vi "demo_1 Single Run.vi"() -> ()   [LabVIEW 2020]
panel:
  out "mtr status":bool caption="电机运行状态"
  in  "microstepping":u16(ring)=32 caption="细分" items=["1 (200)"=1, "2 (400)"=2, "4 (800)"=4, "8 (1600)"=8, "16 (3200)"=16, "32 (6400)"=32]
  in  "speed":u16 caption="转速 (RPM)"
  in  "distance":dbl caption="转动量 (°)"
  in  "direction":u16(ring) caption="旋向" items=["positive", "negative"]
  in  "VISA resource name":refnum<visa-resource-name> caption="VISA资源"
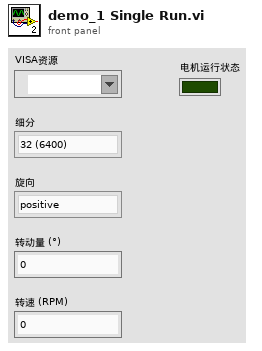
[diagram p1: front panel]
types:
  T1 = cluster{"full step angle":dbl, "microstepping":u16, "start frequency":u16, "stop frequency":u16, "screw pitch":dbl, "distance":dbl, "stop mode":u16, "direction":u16, "speed":u16, "relative / absolute":u16}
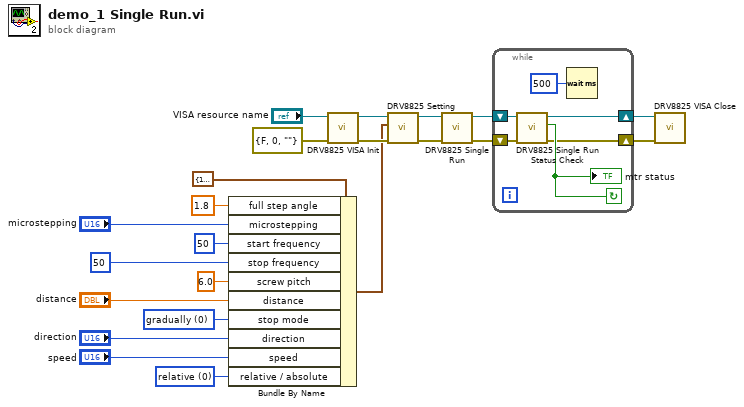
[diagram p0: block diagram]
diagram:
  w12 = u16 0 items=["gradually", "immediately"] ("stop mode")
  w11 = u16 0 items=["relative", "absolute"] ("relative / absolute")
  n1 = Bundle By Name(cluster=T1 {"full step angle"=1.8, "microstepping"=32, "start frequency"=50, "stop frequency"=50, "screw pitch"=360.0, "distance"=0.0, "stop mode"=0, "direction"=0, "speed"=50, "relative / absolute"=0} ("settings"), "full step angle"=1.8, "microstepping"="microstepping", "start frequency"=u16 50, "stop frequency"=u16 50, "screw pitch"=6.0, "distance"="distance", "stop mode"=w12, "direction"="direction", "speed"="speed", "relative / absolute"=w11) -> (w5:T1)
  n2 = call "DRV8825 VISA Init.vi"("error in (no error)"=errorcluster {"status"=FALSE, "code"=0, "source"=""}, "VISA resource name"="VISA resource name") -> ("error out"=w19:errorcluster, "VISA resource name out"=w20:refnum<visa-resource-name>)  [unwired: 8 in]
  n3 = call "DRV8825 Setting.vi"("error in (no error)"=w19, "settings"=w5, "VISA resource name"=w20) -> ("error out"=w17:errorcluster, "VISA resource name out"=w18:refnum<visa-resource-name>)  [unwired: 7 in]
  n4 = call "DRV8825 Single Run.vi"("error in (no error)"=w17, "VISA resource name"=w18) -> ("error out"=w3:errorcluster, "VISA resource name out"=w4:refnum<visa-resource-name>)  [unwired: 8 in]
  n5 = while {
    shift-right: [w24] -> w2
    shift-left: w4 -> [w28]
    shift-right: [w25] -> w1
    shift-left: w3 -> [w27]
    stop <- w26 continue-if-true
    n6 = call "DRV8825 Single Run Status Check.vi"("error in (no error)"=w27, "VISA resource name"=w28) -> ("error out"=w25:errorcluster, "status"=w26:bool, "VISA resource name out"=w24:refnum<visa-resource-name>)  [unwired: 7 in]
    "mtr status" <- w26
    n7 = Wait (ms)(milliseconds to wait=u32 500 ("等待时间（毫秒）")) -> ()  [unwired: 1 out]
  }
  n8 = call "DRV8825 VISA Close.vi"("error in (no error)"=w1, "VISA resource name"=w2) -> ()  [unwired: 9 in, 1 out]
